vi "Read_Electrical_Variables_v2.vi"(8 "error in (no error)":errorcluster, 11 "Modbus master in":refnum<class "Modbus Master.lvclass">) -> (0 "error out":errorcluster, 2 "Variables":sgl[](array[numeric]), 3 "Modbus master out":refnum<class "Modbus Master.lvclass">)   [LabVIEW 2018]
uses:
  <vilib>/Modbus/master/Modbus Master.lvclass
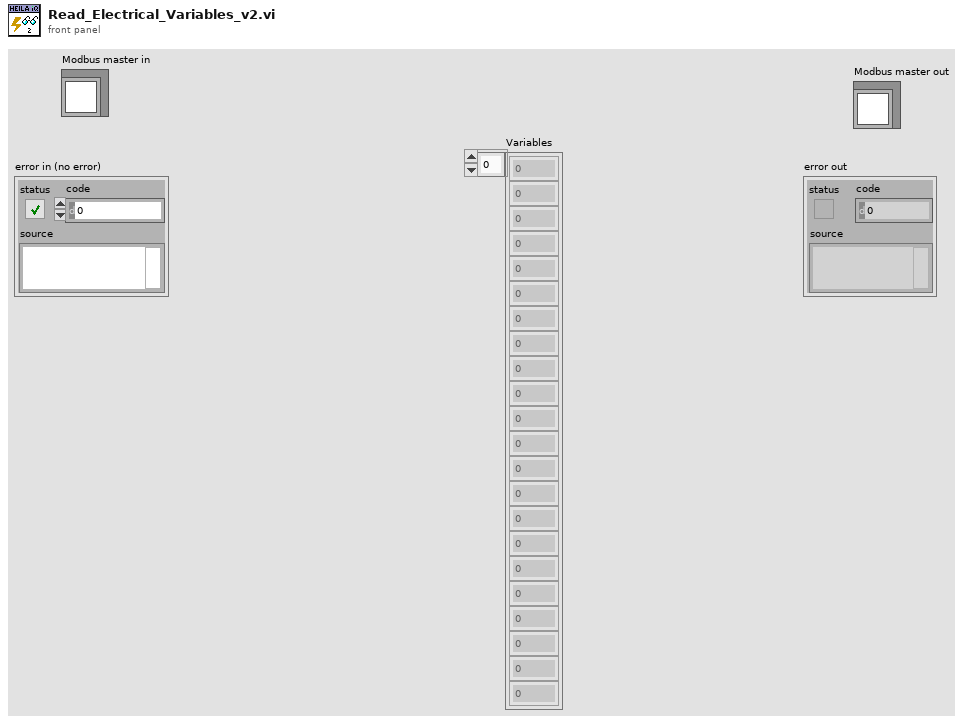
[diagram p1: front panel]
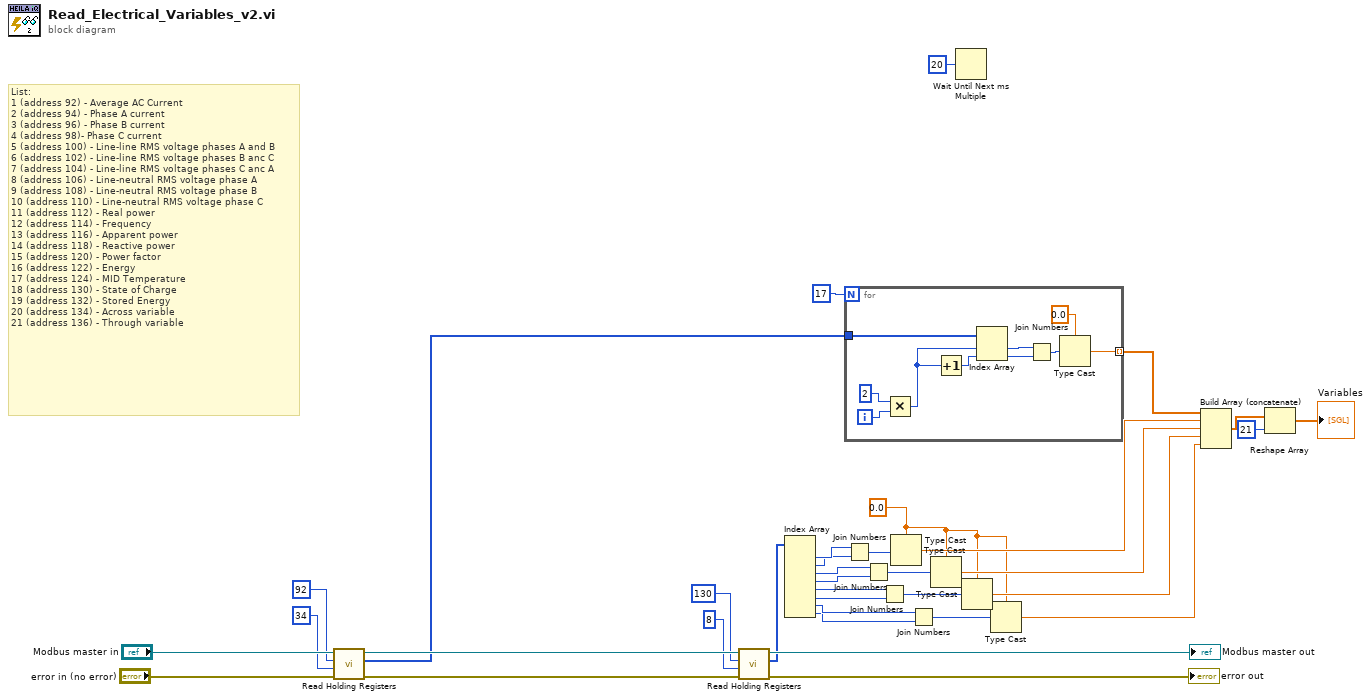
[diagram p0: block diagram]
diagram:
  w3 = sgl 0.0
  # "List:\n1 (address 92) - Average AC Current\n2 (address 94) - Phase A current\n3 (address 96) - Phase B current\n4 (address 98)- Phase C current\n5 (address 100) - Line-line RMS voltage phases A and B\n6 (address 102) - Line-line RMS voltage phases B anc C\n7 (address 104) - Line-line RMS voltage phases C anc A\n8 (address 106) - Line-neutral RMS voltage phase A\n9 (address 108) - Line-neutral RMS voltage phase B\n10 (address 110) - Line-neutral RMS voltage phase C\n11 (address 112) - Real power\n12 (address 114) - Frequency\n13 (address 116) - Apparent power\n14 (address 118) - Reactive power\n15 (address 120) - Power factor\n16 (address 122) - Energy\n17 (address 124) - MID Temperature\n18 (address 130) - State of Charge\n19 (address 132) - Stored Energy\n20 (address 134) - Across variable\n21 (address 136) - Through variable"
  n1 = call-dynamic "Read Holding Registers.vi"("error in (no error)"="error in (no error)", "number of holding registers"=u16 34 ("starting address"), "starting address"=u16 92, "Modbus master in"="Modbus master in") -> ("error out"=w30:errorcluster, "register values"=w20:u16[], "Modbus master out"=w31:refnum<class "Modbus Master.lvclass">)  [unwired: 5 in]
  n2 = call-dynamic "Read Holding Registers.vi"("error in (no error)"=w30, "number of holding registers"=u16 8 ("starting address"), "starting address"=u16 130, "Modbus master in"=w31) -> ("error out"=→"error out":errorcluster, "register values"=w25:u16[], "Modbus master out"=→"Modbus master out":refnum<class "Modbus Master.lvclass">)  [unwired: 5 in]
  n3 = Index Array(array=w25) -> (element #1=w24:u16, element #2=w23:u16, element #3=w14:u16, element #4=w13:u16, element #5=w12:u16, element #6=w11:u16, element #7=w5:u16, element #8=w4:u16)  [unwired: 8 in]
  n4 = for {
    N: 17 -> [_]
    tunnel: [w41] -> w19 mode=indexing
    tunnel: w20 -> [w36]
    i -> [w40]
    n5 = Multiply(x=2, y=w40) -> (x*y=w37:i32)
    n6 = Increment(x=w37) -> (x+1=w38:i32)
    n7 = Index Array(array=w36, index #1=w37, index #2=w38) -> (element #1=w45:u16, element #2=w44:u16)
    n8 = Join Numbers(hi=w45, lo=w44) -> ((hi.lo)=w42:u32)
    n9 = Type Cast(type=sgl 0.0, x=w42) -> (*(type *) &x=w41:sgl)
  }
  n10 = Join Numbers(hi=w24, lo=w23) -> ((hi.lo)=w22:u32)
  n11 = Join Numbers(hi=w14, lo=w13) -> ((hi.lo)=w10:u32)
  n12 = Join Numbers(hi=w12, lo=w11) -> ((hi.lo)=w9:u32)
  n13 = Type Cast(type=w3, x=w22) -> (*(type *) &x=w18:sgl)
  n14 = Join Numbers(hi=w5, lo=w4) -> ((hi.lo)=w6:u32)
  n15 = Type Cast(type=w3, x=w10) -> (*(type *) &x=w8:sgl)
  n16 = Wait Until Next ms Multiple(millisecond multiple=u32 20) -> ()  [unwired: 1 out]
  n17 = Type Cast(type=w3, x=w9) -> (*(type *) &x=w7:sgl)
  n18 = Type Cast(type=w3, x=w6) -> (*(type *) &x=w2:sgl)
  n19 = Build Array (concatenate)(w19, w18, w8, w7, w2) -> (w17:sgl[])
  n20 = Reshape Array(w17, 21 ("dimension size")) -> (→"Variables":sgl[])
